vi "Destroy.vi"   [LabVIEW 2018, in "Toolkit.lvlib" / "Known Hosts.lvclass"]
doc: "Destroys this Known Hosts object and frees the memory allocated within the libssh2lv shared library for the internal linked list. No other VIs within the Known Hosts class should be executed after this VI has completed."
uses:
  Known Hosts.lvclass
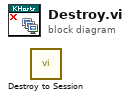
[diagram p0: block diagram]
diagram:
  n1 = call "Destroy to Session.vi"() -> ()  [unwired: 10 in, 2 out]
